vi "Write Pin.vi"(0 "TI in":refnum<class "TI.lvclass">, 5 "Port":dbl, 7 "Pin":dbl, 9 "Value":bool, 11 "error in (no error)":errorcluster) -> (4 "TI out":refnum<class "TI.lvclass">, 15 "error out":errorcluster)   [LabVIEW 2020, in "TI.lvclass"]
doc: "Write Pin es el vi donde se escribe el valor del puerto en binario para que sea recibido por el microcontrolador y pueda encender o apagar el led correspondiente"
uses:
  TI.lvclass
  TI.lvclass/TI.ctl
  4b888cb3-daea-442c-89b9-7bf501ba73cc.vi
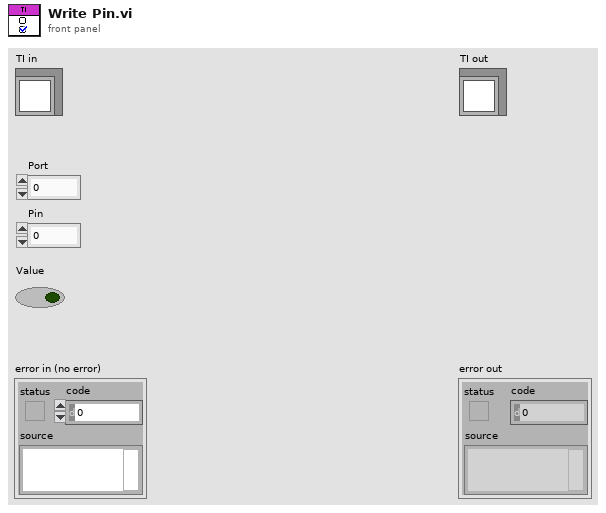
[diagram p1: front panel]
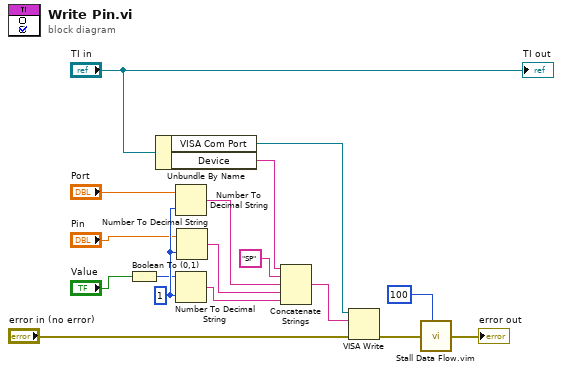
[diagram p0: block diagram]
diagram:
  w9 = i16 1 ("width (-)")
  n1 = Boolean To (0,1)(Boolean="Value") -> (0, 1=w7:i16)
  n2 = Unbundle By Name("TI in") -> ("VISA Com Port"=w16:refnum<visa-resource-name>, "Device"=w14:string)
  n3 = Number To Decimal String(number="Port", width (-)=w9) -> (decimal integer string=w13:string)
  n4 = Number To Decimal String(number=w7, width (-)=w9) -> (decimal integer string=w11:string)
  n5 = Number To Decimal String(number="Pin", width (-)=w9) -> (decimal integer string=w10:string)
  n6 = Concatenate Strings(w14, "SP" ("string"), w13, w10, w11) -> (w15:string)
  n7 = VISA Write(VISA resource name=w16, write buffer=w15, error in (no error)="error in (no error)") -> (error out=w17:errorcluster)  [unwired: 2 out]
  n8 = call "Stall Data Flow.vim"("value in"=w17, "milliseconds to wait"=u32 100) -> ("value out"=→"error out":errorcluster)  [unwired: 1 out]
  "TI out" <- "TI in"
